vi "ServoValueSet.vi"() -> ()   [LabVIEW 2012]
uses:
  <vilib>/FPGAPlugInAG/sbRIO-9636/niLvFpga_Open_sbRIO-9636.vi
  <vilib>/rvi/interface/common/dynamic/niFpgaDynamicAddResources.vi
  <vilib>/rvi/interface/nirviOpenFPGA/nirviOpenFPGA.xnode
  FPGA Bitfiles/NIARC_FPGATarget_FPGACompile_e4XhunWUay0.lvbitx
  FPGA/FPGA Toplevel.vi
panel:
  in  "Angle (deg) Claw":dbl(slide) scale=-90.0..90.0
  in  "Angle (deg) Arm":dbl(slide) scale=-90.0..90.0
  out "error out":errorcluster
  in  "stop":bool
  in  "error in":errorcluster
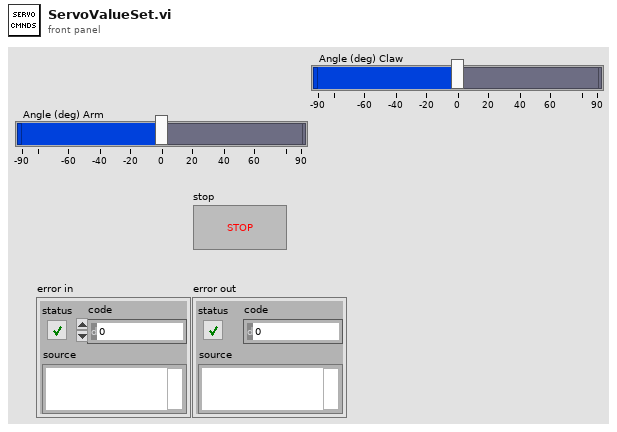
[diagram p1: front panel]
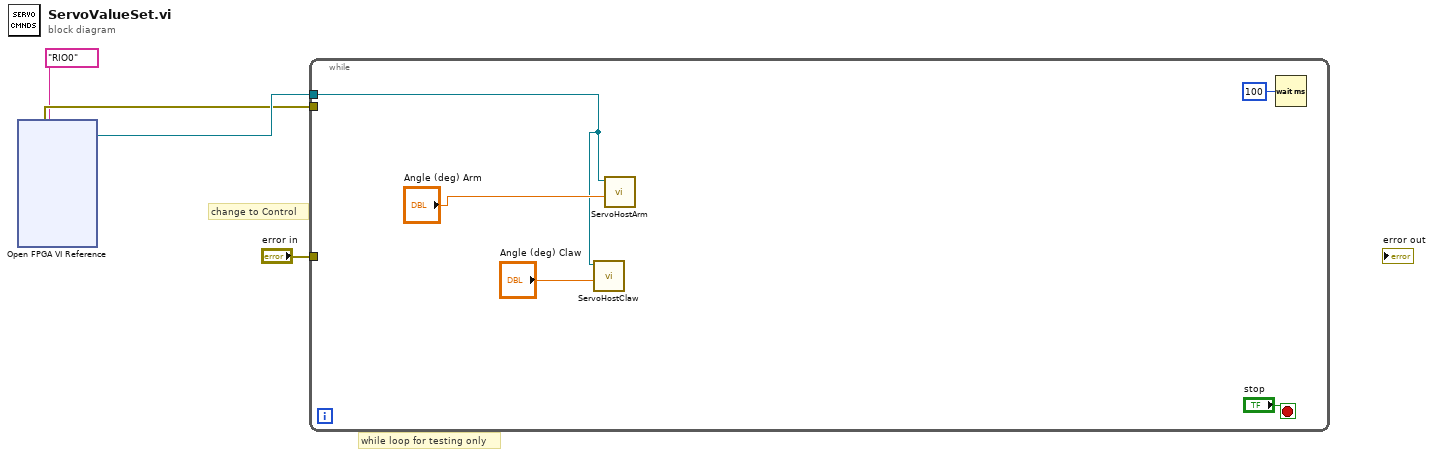
[diagram p0: block diagram]
diagram:
  # "change to Control"
  # "while loop for testing only"
  n1 = xnode "Open FPGA VI Reference"("resource name"=tag "RIO0") -> ("FPGA VI Reference Out"=w3:refnum<k20>, "error out"=w2:errorcluster)  [unwired: 1 in]
  n2 = while {
    tunnel: "error in" -> [_]
    tunnel: w3 -> [w6]
    tunnel: w2 -> [_]
    stop <- "stop" stop-if-true
    n3 = call "ServoHostClaw.vi"("Angle (deg) Claw"="Angle (deg) Claw", "FPGA VI Reference In"=w6) -> ()  [unwired: 8 in, 2 out]
    n4 = call "ServoHostArm.vi"("Angle (deg) Arm"="Angle (deg) Arm", "FPGA VI Reference In"=w6) -> ()  [unwired: 8 in, 2 out]
    n5 = Wait (ms)(milliseconds to wait=u32 100) -> ()  [unwired: 1 out]
  }
